vi "Problem 13.vi"(11 "Huge Ass Number":string="37107287533902102798797998220837590246510135740250\n46376937677490009712648124896970078050417018260538\n74324986199524741059474233309513058123726617309629\n91942213363574161572522430563301811072406154908250\n23067588207539346171171980310421047513778063246676\n89261670696623633820136378418383684178734361726757\n28112879812849979408065481931592621691275889832738\n44274228917432520321923589422876796487670272189318\n47451445736001306439091167216856844588711603153276\n70386486105843025439939619828917593665686757934951\n62176457141856560629502157223196586755079324193331\n649063524627419049291014324458138226633...") -> (3 "Answer":string)   [LabVIEW 2013, in "Problem 13.lvlib"]
uses:
  Problem 13.lvlib
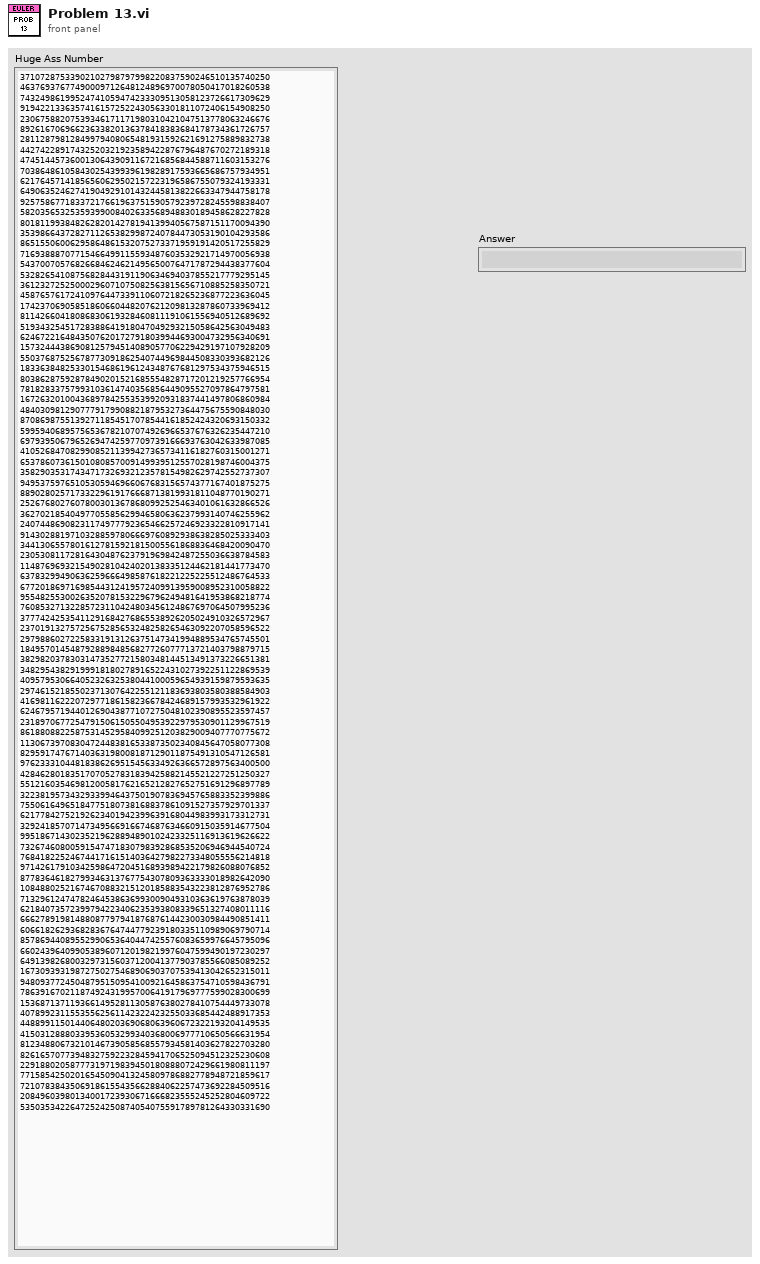
[diagram p1: front panel]
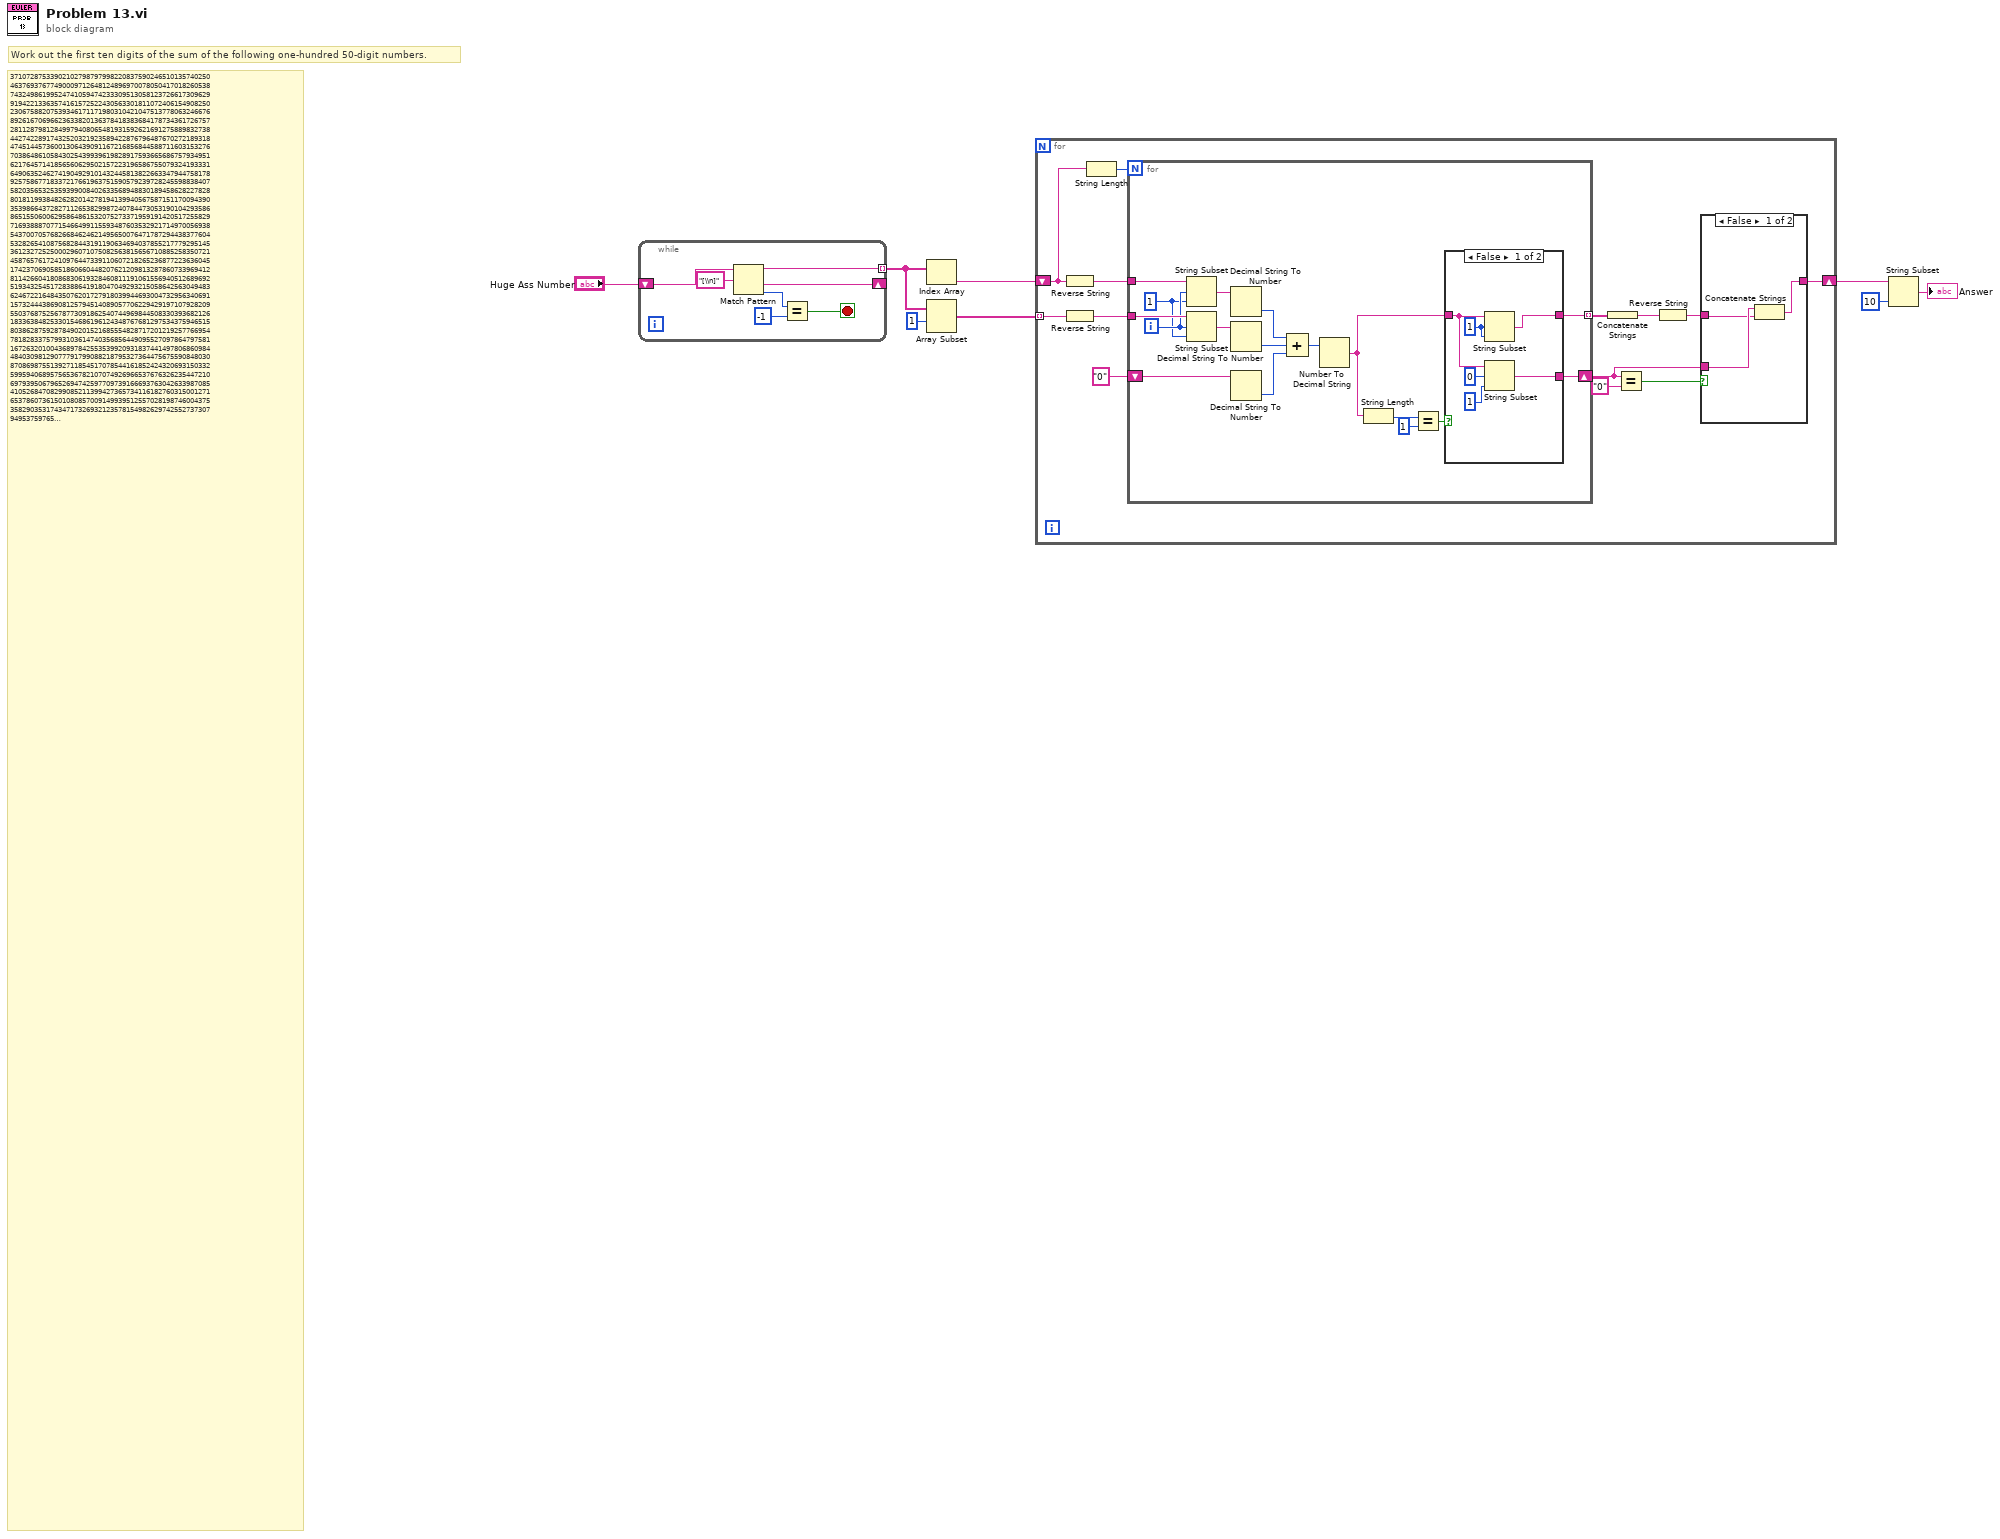
[diagram p0: block diagram]
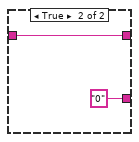
[diagram p3: hidden frame]
diagram:
  # "Work out the first ten digits of the sum of the following one-hundred 50-digit numbers."
  # "37107287533902102798797998220837590246510135740250\n46376937677490009712648124896970078050417018260538\n74324986199524741059474233309513058123726617309629\n91942213363574161572522430563301811072406154908250\n23067588207539346171171980310421047513778063246676\n89261670696623633820136378418383684178734361726757\n28112879812849979408065481931592621691275889832738\n44274228917432520321923589422876796487670272189318\n47451445736001306439091167216856844588711603153276\n70386486105843025439939619828917593665686757934951\n62176457141856560629502157223196586755079324193331\n64906352462741904929101432445813822663347944758178\n92575867718337217661963751590579239728245598838407\n58203565325359399008402633568948830189458628227828\n80181199384826282014278194139940567587151170094390\n35398664372827112653829987240784473..."
  n1 = while {
    shift-right: [w13] -> _
    shift-left: "Huge Ass Number" -> [w14]
    tunnel: [w12] -> w7 mode=indexing
    stop <- w9 stop-if-true
    n2 = Match Pattern(string=w14, regular expression="[\\n]") -> (before substring=w12:string, after substring=w13:string, offset past match=w11:i32)  [unwired: 1 in, 1 out]
    n3 = Equal?(x=w11, y=-1) -> (x = y?=w9:bool)
  }
  n4 = Index Array(array=w7) -> (element=w5:string)  [unwired: 1 in]
  n5 = Array Subset(array=w7, index=1) -> (w4:string[])  [unwired: 1 in]
  n6 = for {
    shift-right: [w17] -> w3
    shift-left: w5 -> [w20]
    tunnel: w4 -> [w28] mode=indexing
    n7 = Reverse String(1:w20) -> (0:w27:string)
    n8 = Reverse String(1:w28) -> (0:w26:string)
    n9 = String Length(string=w20) -> (length=w21:i32)
    n10 = for {
      N: w21 -> [_]
      tunnel: w27 -> [w49]
      tunnel: w26 -> [w48]
      shift-right: [w33] -> w22
      shift-left: "0" -> [w43]
      tunnel: [w35] -> w19 mode=indexing
      i -> [w47]
      w46 = 1 ("length (rest)")
      n11 = String Subset(string=w49, offset (0)=w47, length (rest)=w46) -> (substring=w45:string)
      n12 = String Subset(string=w48, offset (0)=w47, length (rest)=w46) -> (substring=w44:string)
      n13 = Decimal String To Number(string=w45) -> (number=w42:i32)  [unwired: 2 in, 1 out]
      n14 = Decimal String To Number(string=w44) -> (number=w40:i32)  [unwired: 2 in, 1 out]
      n15 = Decimal String To Number(string=w43) -> (number=w41:i32)  [unwired: 2 in, 1 out]
      n16 = Compound Arithmetic op=ADD(w42, w40, w41) -> (w39:i32)
      n17 = Number To Decimal String(number=w39) -> (decimal integer string=w36:string)  [unwired: 1 in]
      n18 = String Length(string=w36) -> (length=w38:i32)
      n19 = Equal?(x=w38, y=1) -> (x = y?=w34:bool)
      n20 = case shown="False" w34 {
        tunnel: w36 -> [w52 w57]
        tunnel: [w50 w57] -> w35
        tunnel: [w53 "0"] -> w33
        frame False {
          w51 = 1 ("offset (0)")
          n21 = String Subset(string=w52, offset (0)=w51, length (rest)=w51) -> (substring=w50:string)
          n22 = String Subset(string=w52, offset (0)=0, length (rest)=1 ("length (rest)")) -> (substring=w53:string)
        }
        frame True {
        }
      }
    }
    n23 = Concatenate Strings(w19) -> (w18:string)
    n24 = Equal?(x=w22, y="0") -> (x = y?=w23:bool)
    n25 = Reverse String(1:w18) -> (0:w16:string)
    n26 = case shown="False" w23 {
      tunnel: [w30 w32] -> w17
      tunnel: w22 -> [w31 _]
      tunnel: w16 -> [w29 w32]
      frame False {
        n27 = Concatenate Strings(w31, w29) -> (w30:string)
      }
      frame True {
      }
    }
  }
  n28 = String Subset(string=w3, length (rest)=10 ("length (rest)")) -> (substring=→"Answer":string)  [unwired: 1 in]
